vi "Parse Qualified Method Name.vi"(11 "Case":string) -> (2 "Method Name":string, 3 "Test Case Class Name":string)   [LabVIEW 2020, in "LUnit Utilities.lvlib"]
uses:
  LUnit Utilities.lvlib
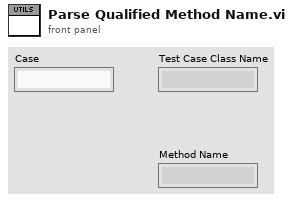
[diagram p1: front panel]
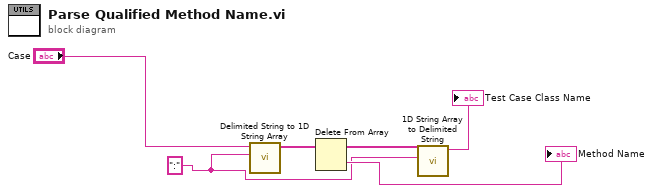
[diagram p0: block diagram]
diagram:
  w4 = ":" ("delimiter")
  n1 = call <vilib>:"Delimited String to 1D String Array.vi"("delimiter"=w4, "delimited string"="Case") -> ("string array"=w2:string[])  [unwired: 9 in]
  n2 = Delete From Array(array=w2) -> (deleted portion=→"Method Name":string, array with subset deleted=w3:string[])  [unwired: 2 in]
  n3 = call <vilib>:"1D String Array to Delimited String.vi"("delimiter"=w4, "string array"=w3) -> ("delimited string"=→"Test Case Class Name":string)  [unwired: 9 in]
